vi "sabertooth packetized build message.vi"(1 "All Data":u8[](array[numeric])=[0, 0, 0, 0], 2 "All Commands":u8[](array[numeric])=[0, 0, 0, 0], 3 "All Addresses":u8[](array[numeric])=[0, 0]) -> (0 "Uart Write Data":string)   [LabVIEW 2018]
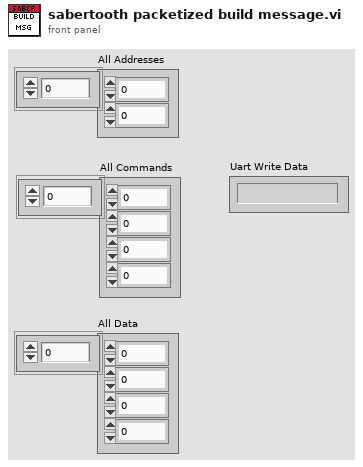
[diagram p1: front panel]
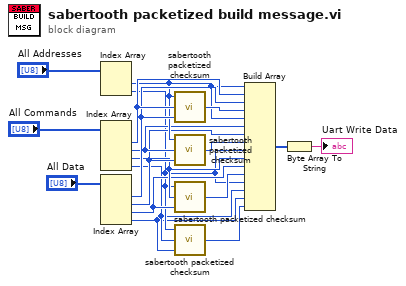
[diagram p0: block diagram]
diagram:
  n1 = Index Array(array="All Addresses") -> (element #1=w11:u8, element #2=w4:u8)  [unwired: 2 in]
  n2 = Index Array(array="All Commands") -> (element #1=w15:u8, element #2=w10:u8, element #3=w7:u8, element #4=w3:u8)  [unwired: 4 in]
  n3 = Index Array(array="All Data") -> (element #1=w14:u8, element #2=w9:u8, element #3=w6:u8, element #4=w2:u8)  [unwired: 4 in]
  n4 = call "sabertooth packetized checksum.vi"("Data"=w14, "Command"=w15, "Address"=w11) -> ("Checksum"=w13:u8)
  n5 = call "sabertooth packetized checksum.vi"("Data"=w9, "Command"=w10, "Address"=w11) -> ("Checksum"=w8:u8)
  n6 = call "sabertooth packetized checksum.vi"("Data"=w6, "Command"=w7, "Address"=w4) -> ("Checksum"=w5:u8)
  n7 = call "sabertooth packetized checksum.vi"("Data"=w2, "Command"=w3, "Address"=w4) -> ("Checksum"=w1:u8)
  n8 = Build Array(w11, w15, w14, w13, w11, w10, w9, w8, w4, w7, w6, w5, w4, w3, w2, w1) -> (w12:u8[])
  n9 = Byte Array To String(unsigned byte array=w12) -> (string=→"Uart Write Data":string)
